vi "mhk_Multi-Function-Synch AI-AO_20103c.vi"() -> ()   [LabVIEW 2010]
doc: "I. Description:\nThis example demonstrates how to continuously acquire and generate data at the same time, synchronized with one another.\n\nII. Instructions for Running:\n1. Select the physical channel to correspond to where your signal is input on the DAQ device. Also, select the corresponding channel for where your signal is being generated.\n2. Enter the minimum and maximum voltage ranges.\nNote: For better accuracy try to match the input range to the expected voltage level of the measured signal.\n3. Set the sample rate of the acquisition.\nNote: The rate should be at least twice as fast as the maximum frequency component of the signal being acquired. \n6. Select the Rate for the generation\n7. Select what type of signal to generate and the amplitude.\nNote: This example requires two DMA channels to run. If your hardware does not support two DMA channels, you need to set the Data Transfer Mechanism property for the Analog Output Task to use \"Interrupts\". The Data Transfer Mechanism property is located in the DAQmx Channel Property hierarchy at:\n\nDAQmx Channel Property Node>>Analog Output>>General Properties>>Advanced>>Data Transfer and Memory>>Data Transfer Mechanism\n\nRefer to your device documentation to determine how many DMA channels are supported for your hardware.\n\nIII. Block Diagram Steps:\n1. Create an analog input voltage channel. Also, create an analog output voltage channel.\n2. Set the rate for the sample clock. Additionally, define the sample mode to be continuous. Also, set the sample clock rate for the signal generation.\n2a. Call the Get Terminal Name with Device Prefix VI. This will take a Task and a terminal and create a properly formatted device + terminal name to use as the source of the Trigger.\n3. Define the parameters for a Digital Edge Start Trigger. Set the Analog output to trigger off the AI Start Trigger. This is an internal trigger signal.\n4. Use the Basic Function Generator VI to create the signal to be generated.\n5. Call the Start VI to arm the two functions. Make sure the analog output is armed before the analog input. This will ensure both will start at the same time.\n6. Read the waveform data in a loop until the user hits the stop button or an error occurs. The Is Task Done? VI is used to check for errors in the Analog Output Task.\n7. Call the Clear VI to Clear the Task\n8. Use the popup dialog box to display an error if any.\n\nIV. I/O Connections Overview:\nMake sure your signal input/output terminals match the Physical Channel I/O controls."
uses:
  <vilib>/Utility/error.llb/DialogType.ctl
  <vilib>/DAQmx/write.llb/DAQmx Write (Analog Wfm 1Chan NSamp).vi
  <vilib>/DAQmx/read.llb/DAQmx Read (Analog 1D Wfm NChan NSamp).vi
  <vilib>/DAQmx/create/channels.llb/DAQmx Create Channel (AI-Voltage-Basic).vi
  <vilib>/DAQmx/configure/timing.llb/DAQmx Timing (Sample Clock).vi
  <vilib>/DAQmx/create/channels.llb/DAQmx Create Channel (AO-Voltage-Basic).vi
  <vilib>/DAQmx/configure/trigger.llb/DAQmx Start Trigger (Digital Edge).vi
  <vilib>/daqmx/miscellaneous.llb/DAQmx Fill In Error Info.vi
  <vilib>/measure/NI_MABase.lvlib
  Program Files (x86)/National Instruments/LabVIEW 2010/resource/objmgr/daqmx.rc
panel:
  in  "# of points to generate":dbl=1000.0
  in  "frequency":dbl=20.0 format="%0.2p"
  in  "offset":dbl format="%0.2p"
  out "Actual Update Generation Rate":dbl=5000.0 format="%0.2f"
  out "Actual Input Rate":dbl=10000.0 format="%0.2f"
  in  "Amplitude":dbl=1.0 format="%0.2p"
  in  "Signal Type":T1(ring)
  in  "rate":dbl=5000.0 caption="Update Generation Rate" format="%0.2f"
  in  "Samples to Read":i32=1000
  in  "minimum value":dbl=-10.0 caption="Output Minimum Value" format="%0.2f"
  in  "maximum value":dbl=10.0 caption="Output Maximum Value" format="%0.2f"
  in  "physical channels":tag="Dev2/ao0" caption="Output Physical Channels"
  in  "Maximum Value":dbl=10.0 caption="Input Maximum Value" format="%0.2f"
  in  "Minimum Value":dbl=-10.0 caption="Input Minimum Value" format="%0.2f"
  in  "Physical Channel":tag="Dev2/ai1:2" caption="Input Physical Channel"
  in  "Rate":dbl=10000.0 caption="Input Rate" format="%0.2f"
  in  "stop":bool
  out "Measurement":waveform(dbl)[](graph)=[{"t0"=timestamp(3386280799.007644 s since 1904-01-01), "dt"=9.999999999999999e-05, "Y"=array[1000 elements], "attributes"=variant("NI_ChannelName"=variant(string "Dev2/ai1"), "NI_UnitDescription"=variant(string "Volts"))}, {"t0"=timestamp(3386280799.0076594 s since 1904-01-01), "dt"=9.999999999999999e-05, "Y"=array[1000 elements], "attributes"=variant("NI_ChannelName"=variant(string "Dev2/ai2"), "NI_UnitDescription"=variant(string "Volts"))}]
  # "For instructions, select Help>>Show Context Help"
  # "Channel Parameters"
  # "Timing Parameters"
  # "Signal Generation"
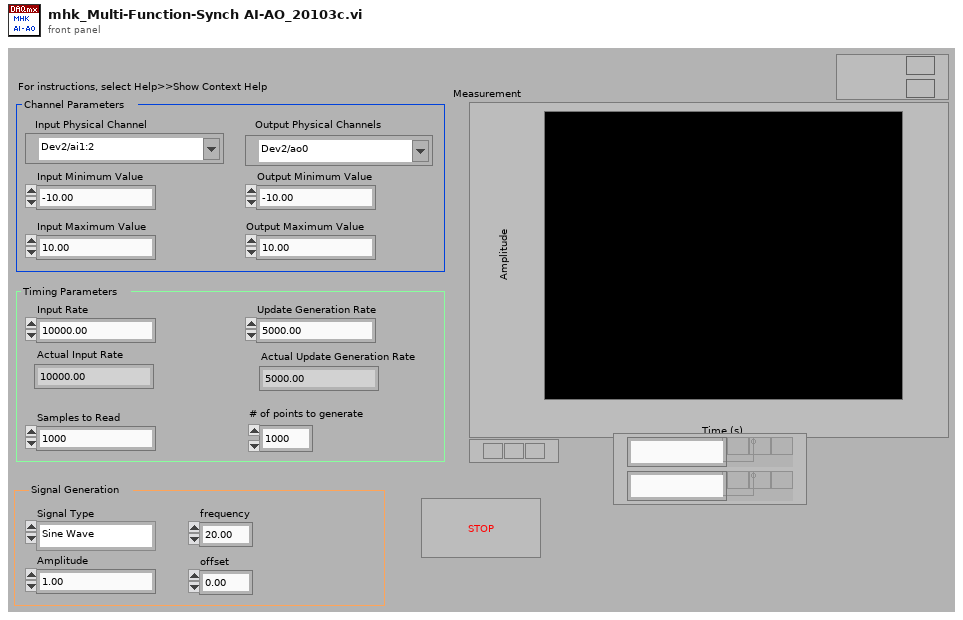
[diagram p1: front panel]
types:
  T1 = enum16{"Sine Wave", "Triangle Wave", "Square Wave", "Sawtooth Wave"}
  T2 = typedef "DialogType.ctl" = u16
  T3 = cluster{"SampClk.Rate":dbl, "# of points to generate":dbl}
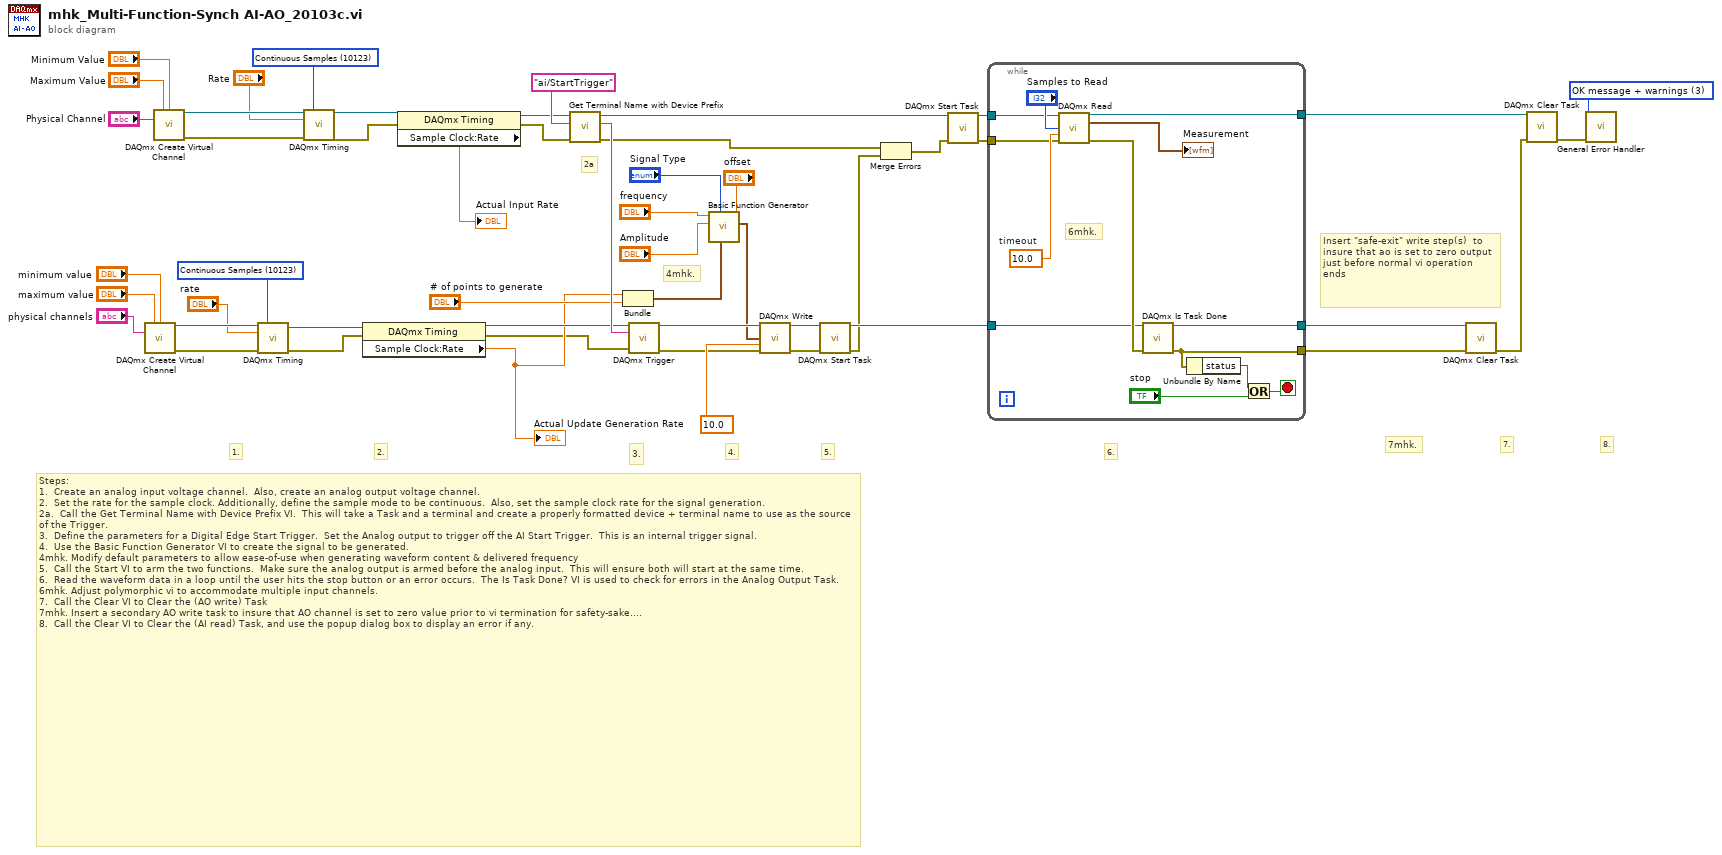
[diagram p0: block diagram]
diagram:
  w31 = T2 3 items=["no dialog", "OK message", "continue or stop message", "OK message + warnings", "continue/stop + warnings"] ("type of dialog (OK msg:1)")
  w42 = 10123 items=["Finite Samples"=10178, "Continuous Samples"=10123] ("sample mode")
  w48 = 10123 items=["Finite Samples"=10178, "Continuous Samples"=10123] ("sample mode")
  # "7mhk."
  # "Insert \"safe-exit\" write step(s)  to insure that ao is set to zero output just before normal vi operation ends"
  # "4mhk."
  # "2a"
  # "6."
  # "3."
  # "4."
  # "8."
  # "5."
  # "7."
  # "Steps: \n1.  Create an analog input voltage channel.  Also, create an analog output voltage channel.\n2.  Set the rate for the sample clock. Additionally, define the sample mode to be continuous.  Also, set the sample clock rate for the signal generation.\n2a.  Call the Get Terminal Name with Device Prefix VI.  This will take a Task and a terminal and create a properly formatted device + terminal name to use as the source of the Trigger.\n3.  Define the parameters for a Digital Edge Start Trigger.  Set the Analog output to trigger off the AI Start Trigger.  This is an internal trigger signal.\n4.  Use the Basic Function Generator VI to create the signal to be generated. \n4mhk. Modify default parameters to allow ease-of-use when generating waveform content & delivered frequency\n5.  Call the Start VI to arm the two functions.  Make sure the analog output is armed before the analog input.  This will ensure both will start at the same time.\n6.  Read the waveform data in a loop until the user hits the stop button or an error occurs.  The Is Task Done? VI is used to check for errors in the Analog Output Task.\n6mhk. Adjust polymorphic vi to accommodate multiple input channels.\n7.  Call the Clear VI to Clear the (AO write) Task\n7mhk. Insert a secondary AO write task to insure that AO channel is set to zero value prior to vi termination for safety-sake....\n8.  Call the Clear VI to Clear the (AI read) Task, and use the popup dialog box to display an error if any."
  # "2."
  # "1."
  n1 = call-poly <vilib>:"DAQmx Create Virtual Channel.vi"("maximum value"="maximum value", "minimum value"="minimum value", "physical channels"="physical channels") -> ("task out"=w41:refnum<k21>, "error out"=w40:errorcluster)  [unwired: 11 in]
  n2 = call-poly <vilib>:"DAQmx Create Virtual Channel.vi"("maximum value"="Maximum Value", "minimum value"="Minimum Value", "physical channels"="Physical Channel") -> ("task out"=w46:refnum<k21>, "error out"=w47:errorcluster)  [unwired: 11 in]
  n3 = call-poly <vilib>:"DAQmx Timing.vi"("task/channels in"=w41, "sample mode"=w42, "rate"="rate", "error in"=w40) -> ("task out"=w23:refnum<k21>, "error out"=w22:errorcluster)  [unwired: 10 in]
  n4 = call-poly <vilib>:"DAQmx Timing.vi"("task/channels in"=w46, "sample mode"=w48, "rate"="Rate", "error in"=w47) -> ("task out"=w15:refnum<k21>, "error out"=w14:errorcluster)  [unwired: 10 in]
  n5 = property class="DAQmx Timing"(reference=w23, error in=w22) -> (reference out=w24:refnum<k21>, error out=w1:errorcluster, "Sample Clock:Rate"=w2:dbl)
  "Actual Update Generation Rate" <- w2
  n6 = property class="DAQmx Timing"(reference=w15, error in=w14) -> (reference out=w13:refnum<k21>, error out=w12:errorcluster, "Sample Clock:Rate"=→"Actual Input Rate":dbl)
  n7 = call "Get Terminal Name with Device Prefix.vi"("error in (no error)"=w12, "Local Terminal Name"="ai/StartTrigger" ("terminal"), "task/channels in"=w13) -> ("error out"=w19:errorcluster, "Terminal Name with Device Prefix"=w25:tag, "task out"=w21:refnum<k21>)  [unwired: 6 in]
  n8 = Bundle("SampClk.Rate"=w2, "# of points to generate"="# of points to generate") -> (w3:T3)  [unwired: 1 in]
  n9 = call-poly <vilib>:"DAQmx Trigger.vi"("task/channels in"=w24, "source"=w25, "error in"=w1) -> ("task out"=w32:refnum<k21>, "error out"=w33:errorcluster)  [unwired: 11 in]
  n10 = call <vilib>:"Basic Function Generator.vi"("offset"="offset", "sampling info"=w3, "signal type"="Signal Type", "amplitude"="Amplitude", "frequency"="frequency") -> ("signal out"=w30:waveform(dbl))  [unwired: 4 in, 2 out]
  n11 = call-poly <vilib>:"DAQmx Write.vi"("task/channels in"=w32, "data"=w30, "timeout"=10.0 ("Wirite Timeout"), "error in"=w33) -> ("task out"=w35:refnum<k21>, "error out"=w34:errorcluster)  [unwired: 9 in, 1 out]
  n12 = call <vilib>:"DAQmx Start Task.vi"("task/channels in"=w35, "error in"=w34) -> ("task out"=w39:refnum<k21>, "error out"=w18:errorcluster)  [unwired: 12 in]
  n13 = Merge Errors(w19, w18) -> (w17:errorcluster)
  n14 = call <vilib>:"DAQmx Start Task.vi"("task/channels in"=w21, "error in"=w17) -> ("task out"=w20:refnum<k21>, "error out"=w16:errorcluster)  [unwired: 12 in]
  n15 = while {
    tunnel: [w64] -> w49
    tunnel: w39 -> [w56]
    tunnel: [w55] -> w38
    tunnel: w20 -> [w54]
    tunnel: w16 -> [w53]
    tunnel: [w52] -> w10
    stop <- w61 stop-if-true
    w62 = 10.0  # timeout
    # "6mhk."
    n16 = call-poly <vilib>:"DAQmx Read.vi"("task/channels in"=w54, "number of samples per channel"="Samples to Read", "timeout"=w62, "error in"=w53) -> ("task out"=w64:refnum<k21>, "data"=→"Measurement":waveform(dbl)[], "error out"=w57:errorcluster)  [unwired: 9 in]
    n17 = call <vilib>:"DAQmx Is Task Done.vi"("task/channels in"=w56, "error in"=w57) -> ("task out"=w55:refnum<k21>, "error out"=w52:errorcluster)  [unwired: 11 in, 1 out]
    n18 = Unbundle By Name(w52) -> ("status"=w58:bool)
    n19 = Or(x=w58, y="stop") -> (x .or. y?=w61:bool)
  }
  n20 = call <vilib>:"DAQmx Clear Task.vi"("task in"=w38, "error in"=w10) -> ("error out"=w9:errorcluster)  [unwired: 13 in]
  n21 = call <vilib>:"DAQmx Clear Task.vi"("task in"=w49, "error in"=w9) -> ("error out"=w8:errorcluster)  [unwired: 13 in]
  n22 = call <vilib>:"General Error Handler.vi"("type of dialog (OK msg:1)"=w31, "error in (no error)"=w8) -> ()  [unwired: 9 in, 5 out]
